vi "Derivative.vi"() -> ()   [LabVIEW 2013]
uses:
  <vilib>/Analysis/3filter.llb/Filter Passband Type.ctl
  <vilib>/Analysis/3filter.llb/Butterworth Filter (DBL).vi
  <vilib>/Analysis/NI_AALBase.lvlib
panel:
  out "Waveform Graph":dbl[](graph)
  out "Derivative":dbl[](array[numeric])
  out "Array in":dbl[](array[numeric])
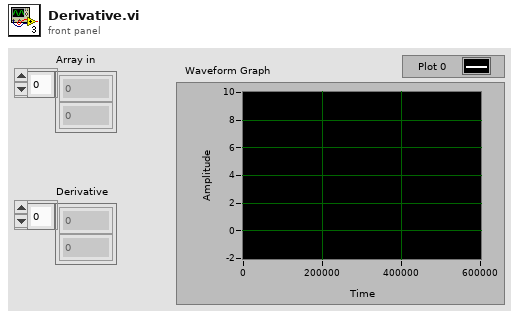
[diagram p1: front panel]
types:
  T1 = enum16{"open", "open or create", "create or replace", "create", "open (read-only)"}
  T2 = typedef "NI_AALBase.lvlib/Filter Passband Type.ctl" = enum32{"Lowpass", "Highpass", "Bandpass", "Bandstop"}
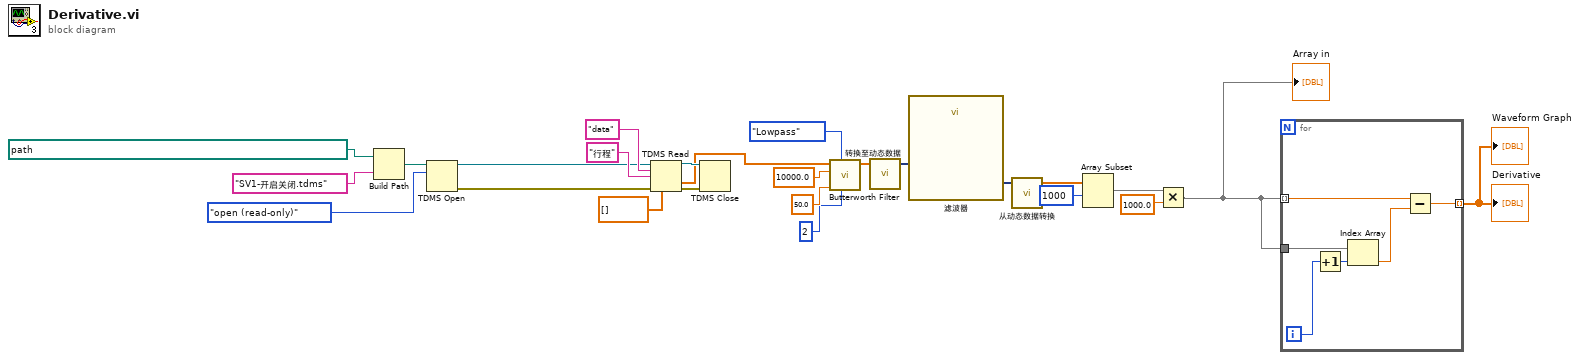
[diagram p0: block diagram]
diagram:
  n1 = Build Path(base path=path "C:/Users/Xiang MU/Desktop/实验文件夹/DR96-03-5/SV1", name or relative path="SV1-开启关闭.tdms") -> (appended path=w7:path)
  n2 = TDMS Open(10:T1."open (read-only)" ("operation (0:open)"), 11:w7) -> (0:w8:errorcluster, 3:w9:refnum<k34>)  [unwired: 5 in]
  n3 = TDMS Read(0:w9, 5:"data" ("组名称输入"), 7:"行程" ("组名称输入"), 11:w8, 12:dbl[] []) -> (4:w21:refnum<k34>, 10:w5:dbl[], 15:w22:errorcluster)  [unwired: 3 in, 3 out]
  n4 = TDMS Close(8:w22, 11:w21) -> ()  [unwired: 2 out]
  n5 = call-poly <vilib>:"Butterworth Filter.vi"("order"=2, "filter type"=Filter_Passband_Type."Lowpass", "low cutoff freq: fl"=50.0, "sampling freq: fs"=10000.0, "X"=w5) -> ("Filtered X"=w16:dbl[])  [unwired: 3 in, 1 out]
  n6 = call "转换至动态数据"("Array"=w16) -> ("Dynamic Data Type"=w14:dynamicdata)  [unwired: 3 in]
  n7 = call "滤波器"("Signal"=w14) -> ("Filtered Signal"=w13:dynamicdata)  [unwired: 9 in, 1 out]
  n8 = call "从动态数据转换"("Dynamic Data Type"=w13) -> ("Array"=w12:dbl[])  [unwired: 3 in]
  n9 = Array Subset(array=w12, index=1000 ("索引")) -> (w10:dbl[])  [unwired: 1 in]
  n10 = Multiply(x=w10, y=1000.0) -> (x*y=w4:dbl[])
  "Array in" <- w4
  n11 = for {
    tunnel: w4 -> [w30]
    tunnel: w4 -> [w29] mode=indexing
    tunnel: [w26] -> w1 mode=indexing
    i -> [w27]
    n12 = Increment(x=w27) -> (x+1=w28:i32)
    n13 = Index Array(array=w30, index=w28) -> (element=w31:dbl)
    n14 = Subtract(x=w29, y=w31) -> (x-y=w26:dbl)
  }
  "Derivative" <- w1
  "Waveform Graph" <- w1
